vi "PCO_GetColorSettings.vi"(8 "error in (no error)":errorcluster {"code" format="%x"}, 11 "ph":u64) -> (0 "error out":errorcluster {"code" format="%x"}, 1 "strColorSet":T1, 2 "ErrorMessage":i32 format="%x", 3 "ph out":u64)   [LabVIEW 2019, in "SDK.lvlib" / "SpecialCommandsDimax_HDSDI.lvlib"]
doc: "<b>Description:</b>\nGets the current color convert parameters of the camera.\n\n<b>Supported camera type:</b>\npco.dimax with HD-SDI interface\n\n<b>Descriptor dependency:</b>\nNone"
uses:
  SpecialCommandsDimax_HDSDI.lvlib
  Structures/Structures.lvlib
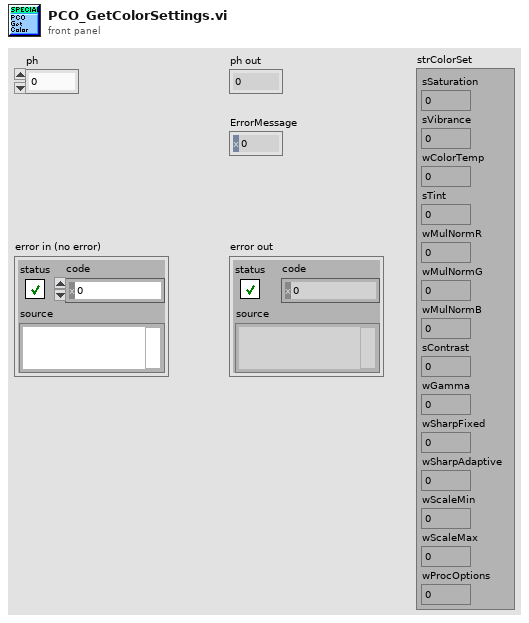
[diagram p1: front panel]
types:
  T1 = cluster{"sSaturation":i16, "sVibrance":i16, "wColorTemp":u16, "sTint":i16, "wMulNormR":u16, "wMulNormG":u16, "wMulNormB":u16, "sContrast":i16, "wGamma":u16, "wSharpFixed":u16, "wSharpAdaptive":u16, "wScaleMin":u16, "wScaleMax":u16, "wProcOptions":u16}
  T2 = cluster{"wSize":u16, "sSaturation":i16, "sVibrance":i16, "wColorTemp":u16, "sTint":i16, "wMulNormR":u16, "wMulNormG":u16, "wMulNormB":u16, "sContrast":i16, "wGamma":u16, "wSharpFixed":u16, "wSharpAdaptive":u16, "wScaleMin":u16, "wScaleMax":u16, "wProcOptions":u16, "ZZwDummy":cluster{u16, u16, u16, u16, u16, u16, u16, u16, u16, u16, u16, u16, u16, u16, u16, u16, u16, u16, u16, u16, u16, u16, u16, u16, u16, u16, u16, u16, u16, u16, u16, u16, u16, u16, u16, u16, u16, u16, u16, u16, u16, u16, u16, u16, u16, u16, u16, u16, u16, u16, u16, u16, u16, u16, u16, u16, u16, u16, u16, u16, u16, u16, u16, u16, u16, u16, u16, u16, u16, u16, u16, u16, u16, u16, u16, u16, u16, u16, u16, u16, u16, u16, u16, u16, u16, u16, u16, u16, u16, u16, u16, u16, u16}}
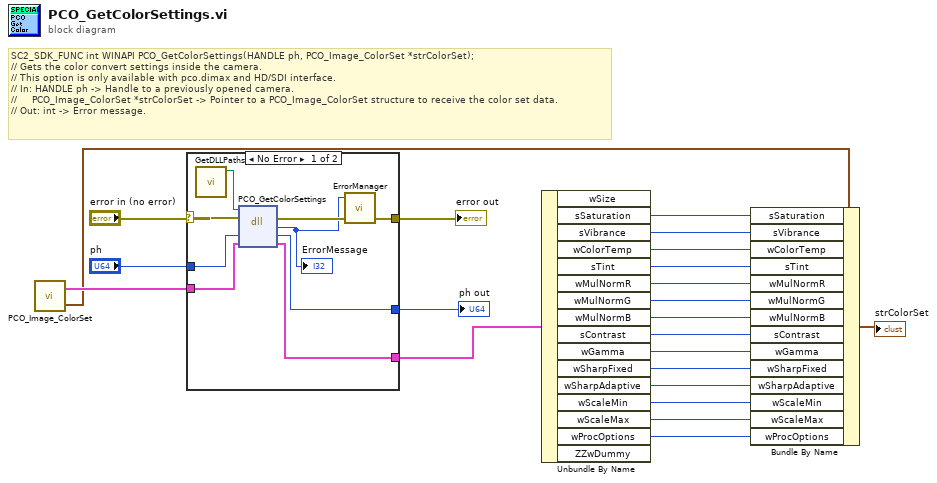
[diagram p0: block diagram]
diagram:
  # "SC2_SDK_FUNC int WINAPI PCO_GetColorSettings(HANDLE ph, PCO_Image_ColorSet *strColorSet);\n// Gets the color convert settings inside the camera.\n// This option is only available with pco.dimax and HD/SDI interface.\n// In: HANDLE ph -> Handle to a previously opened camera.\n//     PCO_Image_ColorSet *strColorSet -> Pointer to a PCO_Image_ColorSet structure to receive the color set data.\n// Out: int -> Error message."
  n1 = call "PCO_Image_ColorSet.vi"() -> ("PCO_Image_ColorSet"=w16:T1, "PCO_Image_ColorSet_Raw"=w18:T2)  [unwired: 4 in, 2 out]
  n2 = case shown="No Error" "error in (no error)" {
    selector: "error in (no error)" -> [w27 w32]
    tunnel: "ph" -> [w31 w33]
    tunnel: [w30 w33] -> w21
    tunnel: w18 -> [w29 w34]
    tunnel: [w28 w34] -> w17
    tunnel: [w26 w32] -> w20
    frame No Error {
      n3 = call "GetDLLPaths.vi"() -> ("SC2_Cam_Path"=w23:path)  [unwired: 9 in, 2 out]
      n4 = dll-call lib="?" fn="PCO_GetColorSettings"(path in=w23, error in=w27, "ph"=w31, "strColorSet"=w29) -> (error out=w25:errorcluster, "return type"=w24:i32, "ph"=w30:u64, "strColorSet"=w28:T2)  [unwired: 1 in, 1 out]
      "ErrorMessage" <- w24
      n5 = call "ErrorManager.vi"("error in (no error)"=w25, "error code"=w24) -> ("error out"=w26:errorcluster)  [unwired: 3 in]
    }
    frame Error {
    }
  }
  "ph out" <- w21
  "error out" <- w20
  n6 = Unbundle By Name(w17) -> ("sSaturation"=w15:i16, "sVibrance"=w14:i16, "wColorTemp"=w13:u16, "sTint"=w12:i16, "wMulNormR"=w11:u16, "wMulNormG"=w10:u16, "wMulNormB"=w9:u16, "sContrast"=w8:i16, "wGamma"=w7:u16, "wSharpFixed"=w6:u16, "wSharpAdaptive"=w5:u16, "wScaleMin"=w4:u16, "wScaleMax"=w3:u16, "wProcOptions"=w2:u16)  [unwired: 2 out]
  n7 = Bundle By Name(cluster=w16, "sSaturation"=w15, "sVibrance"=w14, "wColorTemp"=w13, "sTint"=w12, "wMulNormR"=w11, "wMulNormG"=w10, "wMulNormB"=w9, "sContrast"=w8, "wGamma"=w7, "wSharpFixed"=w6, "wSharpAdaptive"=w5, "wScaleMin"=w4, "wScaleMax"=w3, "wProcOptions"=w2) -> (→"strColorSet":T1)
